vi "Create_PMT_Dir_Gain.vi"(0 "Test":string, 1 "Run":string, 2 "Folder name":string, 3 "PMTs":string[](array[string])) -> (7 "Paths":path[](array[path]))   [LabVIEW 2019]
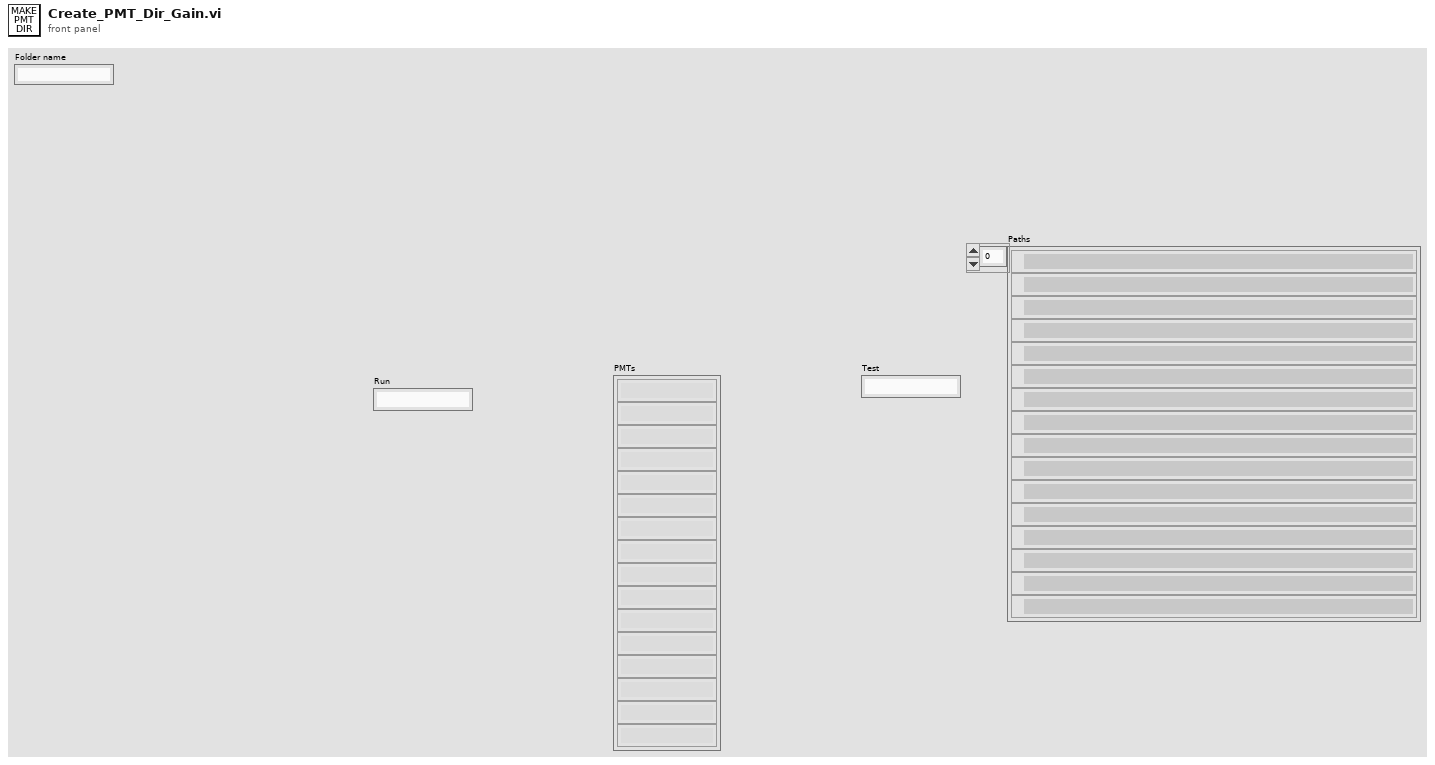
[diagram p1: front panel]
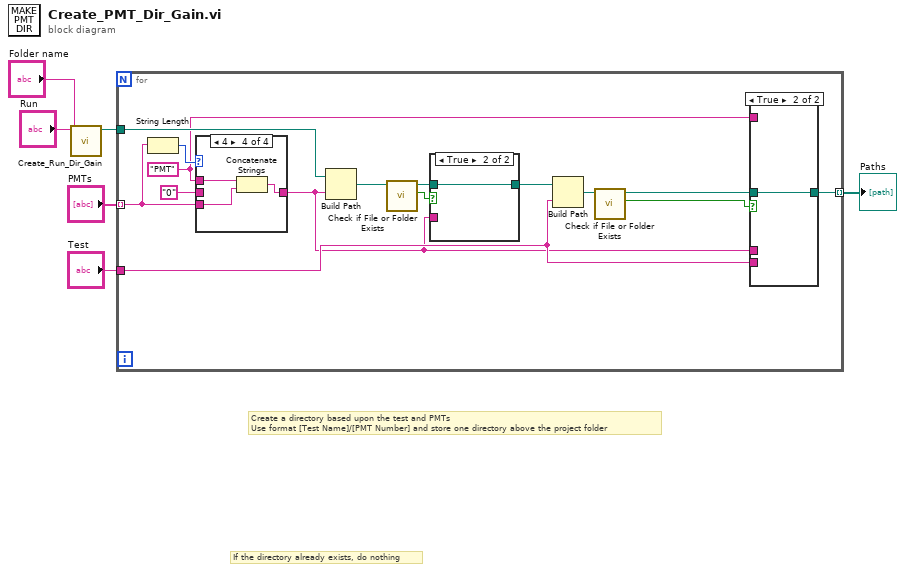
[diagram p0: block diagram]
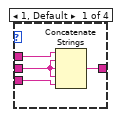
[diagram p2: hidden frame]
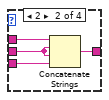
[diagram p3: hidden frame]
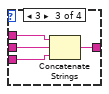
[diagram p4: hidden frame]
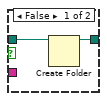
[diagram p5: hidden frame]
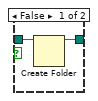
[diagram p6: hidden frame]
diagram:
  # "If the directory already exists, do nothing"
  # "Create a directory based upon the test and PMTs\nUse format [Test Name]/[PMT Number] and store one directory above the project folder"
  n1 = call "Create_Run_Dir_Gain.vi"("Folder name"="Folder name", "Run"="Run") -> ("dup path"=w2:path)  [unwired: 9 in]
  n2 = for {
    tunnel: "PMTs" -> [w10] mode=indexing
    tunnel: w2 -> [w21]
    tunnel: "Test" -> [w8]
    tunnel: [w13] -> w4 mode=indexing
    w11 = "PMT" ("string")
    n3 = String Length(string=w10) -> (length=w12:i32)
    n4 = case shown="4" w12 {
      tunnel: w11 -> [w25 w28 w33 w36]
      tunnel: w10 -> [w23 w26 w31 w35]
      tunnel: [w24 w29 w30 w34] -> w7
      tunnel: "0" ("string") -> [w22 w27 w32 _]
      frame 1, Default {
        n5 = Concatenate Strings(w25, w22, w22, w22, w23) -> (w24:string)
      }
      frame 2 {
        n6 = Concatenate Strings(w28, w27, w27, w26) -> (w29:string)
      }
      frame 3 {
        n7 = Concatenate Strings(w33, w32, w31) -> (w30:string)
      }
      frame 4 {
        n8 = Concatenate Strings(w36, w35) -> (w34:string)
      }
    }
    n9 = Build Path(base path=w21, name or relative path=w7) -> (appended path=w17:path)
    n10 = call <vilib>:"Check if File or Folder Exists.vi"("path"=w17) -> ("file or folder exists?"=w16:bool, "dup path"=w15:path)  [unwired: 8 in, 1 out]
    n11 = case shown="True" w16 {
      tunnel: w15 -> [w38 w39]
      tunnel: [w37 w39] -> w14
      tunnel: w7 -> [_ _]
      frame False {
        n12 = Create Folder(path (use dialog)=w38) -> (created path=w37:path)  [unwired: 2 in, 2 out]
      }
      frame True {
      }
    }
    n13 = Build Path(base path=w14, name or relative path=w8) -> (appended path=w20:path)
    n14 = call <vilib>:"Check if File or Folder Exists.vi"("path"=w20) -> ("file or folder exists?"=w19:bool, "dup path"=w18:path)  [unwired: 8 in, 1 out]
    n15 = case shown="True" w19 {
      tunnel: w18 -> [w41 w42]
      tunnel: [w40 w42] -> w13
      tunnel: w8 -> [_ _]
      tunnel: w11 -> [_ _]
      tunnel: w7 -> [_ _]
      frame False {
        n16 = Create Folder(path (use dialog)=w41) -> (created path=w40:path)  [unwired: 2 in, 2 out]
      }
      frame True {
      }
    }
  }
  "Paths" <- w4
